vi "START IT!.vi"() -> ()   [LabVIEW 2014]
doc: "Launches all the software required for data acquisition."
uses:
  Start all VIs Globals.vi
panel:
  in  "Stop":bool
  in  "Username:":string
  in  "Existing File Location:":path
  in  "Save this session's\n      parameters?":bool
  in  "Load existing file?":bool
  out "Starting Module Number:":u32(slide) scale=0.0..6.0
  out "Status":string="Ready"
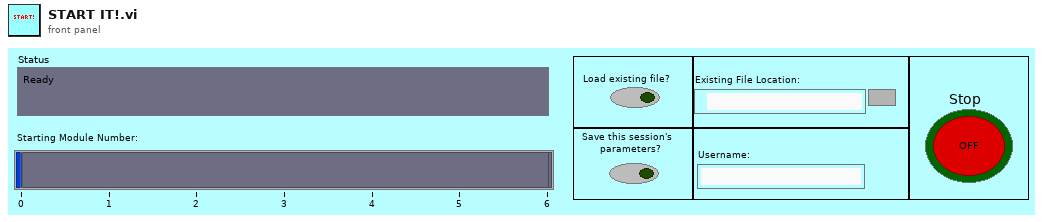
[diagram p1: front panel]
types:
  T1 = enum32{"Invalid", "Standard", "Closed", "Hidden", "Minimized", "Maximized"}
  T2 = enum32{"Bad", "Idle", "Run top level", "Running"}
  T3 = cluster{"VI Name":string, "Location":enum16{"TIRF Lock", "Camera & Acquisition VIs", "Stage Control", "Shutter Control"}, "Run?":bool, "Minimized?":bool, "Subdirectory (w trailing \"/\")":string}[]
  T4 = cluster{"Shutter Control":path, "Stage Control":path, "Camera & Acquisition VIs":path, "TIRF Lock":path}
  T5 = enum16{"TIRF Lock", "Camera & Acquisition VIs", "Stage Control", "Shutter Control"}
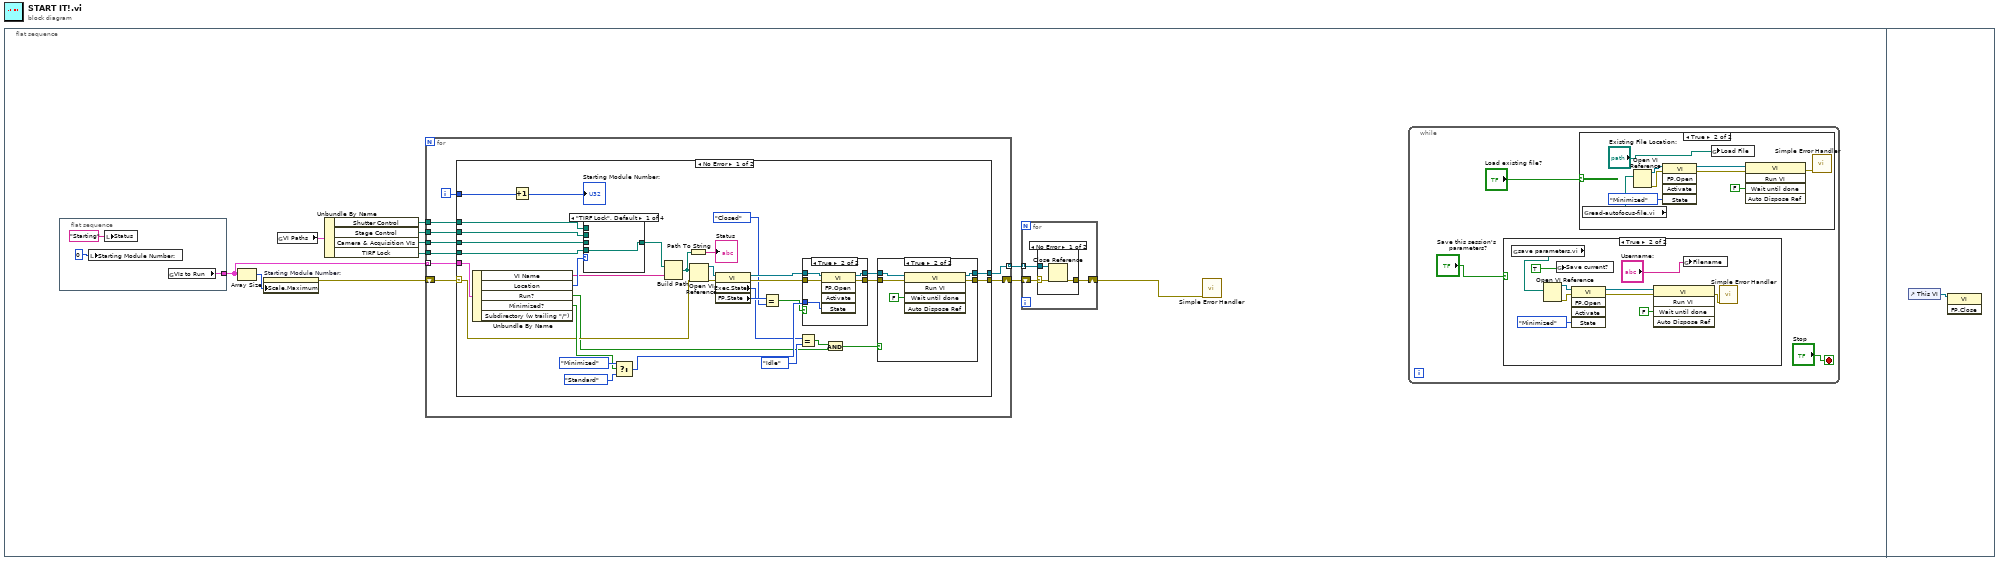
[diagram p0: block diagram]
diagram:
  n1 = flat-sequence {
    frame #0 {
      n2 = flat-sequence {
        tunnel: [w36] -> w2
        frame #0 {
          n3 = local write "Starting Module Number:"(0) -> ()
          n4 = local write "Status"("Starting") -> ()
          n5 = global read "Start all VIs Globals.vi" "VIs to Run"() -> (w36:T3)
        }
      }
      n6 = Array Size(array=w2) -> (size(s)=w3:i32)
      n7 = property on="Starting Module Number:" class="Slide (strict)"("Scale.Maximum"=w3) -> (error out=w4:errorcluster)  [unwired: 2 in, 1 out]
      n8 = global read "Start all VIs Globals.vi" "VI Paths"() -> (w11:T4)
      n9 = Unbundle By Name(w11) -> ("Shutter Control"=w10:path, "Stage Control"=w9:path, "Camera & Acquisition VIs"=w8:path, "TIRF Lock"=w7:path)
      n10 = for {
        tunnel: w10 -> [w51]
        tunnel: w9 -> [w50]
        tunnel: w8 -> [w49]
        tunnel: w7 -> [w48]
        tunnel: w2 -> [w52] mode=indexing
        tunnel: [w47] -> w6 mode=indexing
        shift-right: [w46] -> w5
        shift-left: w4 -> [w45]
        i -> [w44]
        n11 = case shown="No Error" w45 {
          selector: w45 -> [w73 w104]
          tunnel: w52 -> [w85 _]
          tunnel: w51 -> [w83 _]
          tunnel: w50 -> [w82 _]
          tunnel: w49 -> [w81 _]
          tunnel: w48 -> [w80 _]
          tunnel: [w54 _] -> w47
          tunnel: [w53 w104] -> w46
          tunnel: w44 -> [w71 _]
          frame No Error {
            n12 = Unbundle By Name(w85) -> ("VI Name"=w78:string, "Location"=w84:T5, "Run?"=w58:bool, "Minimized?"=w75:bool)  [unwired: 1 out]
            n13 = Increment(x=w71) -> (x+1=→"Starting Module Number:":i32)
            n14 = case shown="\"TIRF Lock\", Default" w84 {
              tunnel: w83 -> [_ _ _ w103]
              tunnel: w82 -> [_ _ w102 _]
              tunnel: w81 -> [_ w101 _ _]
              tunnel: w80 -> [w100 _ _ _]
              tunnel: [w100 w101 w102 w103] -> w79
              frame "TIRF Lock", Default {
              }
              frame "Camera & Acquisition VIs" {
              }
              frame "Stage Control" {
              }
              frame "Shutter Control" {
              }
            }
            n15 = Select(t=T1."Minimized" ("State"), s=w75, f=T1."Standard" ("State")) -> (s? t:f=w74:T1)
            n16 = Build Path(base path=w79, name or relative path=w78) -> (appended path=w69:path)
            n17 = Path To String(path=w69) -> (string=→"Status":string)
            n18 = Open VI Reference(vi path=w69, error in (no error)=w73) -> (vi reference=w67:refnum<vi>, error out=w68:errorcluster)  [unwired: 4 out]
            n19 = property class="VI"(reference=w67, error in=w68) -> (reference out=w65:refnum<vi>, error out=w66:errorcluster, "Exec.State"=w61:T2, "FP.State"=w64:T1)
            n20 = Equal?(x=w64, y=T1."Closed" ("State")) -> (x = y?=w62:bool)
            n21 = Equal?(x=w61, y=T2."Idle") -> (x = y?=w59:bool)
            n22 = case shown="True" w62 {
              tunnel: w65 -> [w93 w99]
              tunnel: w66 -> [w94 w98]
              tunnel: w74 -> [_ w97]
              tunnel: [w93 w96] -> w55
              tunnel: [w94 w95] -> w56
              frame False {
              }
              frame True {
                n23 = invoke class="VI" method="FP.Open"(reference=w99, error in=w98, "State"=w97) -> (reference out=w96:refnum<vi>, error out=w95:errorcluster)  [unwired: 2 in, 3 out]
              }
            }
            n24 = And(x=w59, y=w58) -> (x .and. y?=w57:bool)
            n25 = case shown="True" w57 {
              tunnel: w56 -> [w87 w90]
              tunnel: w55 -> [w86 w91]
              tunnel: [w86 w89] -> w54
              tunnel: [w87 w88] -> w53
              frame False {
              }
              frame True {
                n26 = invoke class="VI" method="Run VI"(reference=w91, error in=w90, "Wait until done"=FALSE ("Wait Until Done")) -> (reference out=w89:refnum<vi>, error out=w88:errorcluster)  [unwired: 2 in, 3 out]
              }
            }
          }
          frame Error {
          }
        }
      }
      n27 = for {
        tunnel: w6 -> [w39] mode=indexing
        shift-right: [w38] -> w1
        shift-left: w5 -> [w37]
        n28 = case shown="No Error" w37 {
          selector: w37 -> [w42 w43]
          tunnel: w39 -> [w41 _]
          tunnel: [w40 w43] -> w38
          frame No Error {
            n29 = Close Reference(reference=w41, error in (no error)=w42) -> (error out=w40:errorcluster)
          }
          frame Error {
          }
        }
      }
      n30 = call <vilib>:"Simple Error Handler.vi"("error in (no error)"=w1) -> ()  [unwired: 4 in, 5 out]
      n31 = while {
        stop <- "Stop" stop-if-true
        n32 = case shown="True" "Save this session's\n      parameters?" {
          frame False {
          }
          frame True {
            n33 = global read "Start all VIs Globals.vi" "save parameters.vi"() -> (w18:path)
            n34 = Open VI Reference(vi path=w18) -> (vi reference=w20:refnum<vi>, error out=w19:errorcluster)  [unwired: 1 in, 4 out]
            n35 = global write "Start all VIs Globals.vi" "Save current?"(TRUE) -> ()
            n36 = invoke class="VI" method="FP.Open"(reference=w20, error in=w19, "State"=T1."Minimized") -> (reference out=w22:refnum<vi>, error out=w23:errorcluster)  [unwired: 2 in, 3 out]
            n37 = invoke class="VI" method="Run VI"(reference=w22, error in=w23, "Wait until done"=FALSE ("Wait Until Done")) -> (error out=w21:errorcluster)  [unwired: 2 in, 4 out]
            n38 = global write "Start all VIs Globals.vi" "Filename"("Username:") -> ()
            n39 = call <vilib>:"Simple Error Handler.vi"("error in (no error)"=w21) -> ()  [unwired: 4 in, 5 out]
          }
        }
        n40 = case shown="True" "Load existing file?" {
          frame False {
          }
          frame True {
            n41 = global read "Start all VIs Globals.vi" "read-autofocus-file.vi"() -> (w27:path)
            n42 = Open VI Reference(vi path=w27) -> (vi reference=w28:refnum<vi>, error out=w29:errorcluster)  [unwired: 1 in, 4 out]
            n43 = invoke class="VI" method="FP.Open"(reference=w28, error in=w29, "State"=T1."Minimized") -> (reference out=w31:refnum<vi>, error out=w32:errorcluster)  [unwired: 2 in, 3 out]
            n44 = global write "Start all VIs Globals.vi" "Load File"("Existing File Location:") -> ()
            n45 = invoke class="VI" method="Run VI"(reference=w31, error in=w32, "Wait until done"=FALSE ("Wait Until Done")) -> (error out=w30:errorcluster)  [unwired: 2 in, 4 out]
            n46 = call <vilib>:"Simple Error Handler.vi"("error in (no error)"=w30) -> ()  [unwired: 4 in, 5 out]
          }
        }
      }
    }
    frame #1 {
      n47 = control-ref of="This VI"() -> (w105:refnum<vi>)
      n48 = invoke class="VI" method="FP.Close"(reference=w105) -> ()  [unwired: 2 in, 3 out]
    }
  }
